vi "SetupDefault.vi"(8 "error in (no error)":errorcluster, 10 "Alias":string, 11 "SpecA_ESA in":refnum<class "SpecA_ESA.lvclass">) -> (0 "error out":errorcluster, 3 "SpecA_ESA out":refnum<class "SpecA_ESA.lvclass">)   [LabVIEW 2014, in "SpecA_ESA.lvclass"]
uses:
  SpecA_ESA.lvclass
  SpecA_ESA.lvclass/SpecA_ESA.ctl
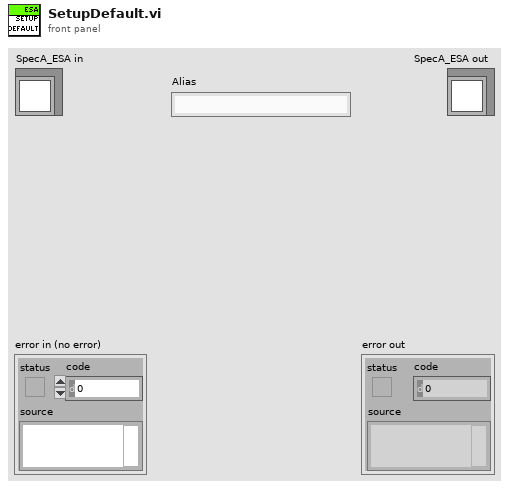
[diagram p1: front panel]
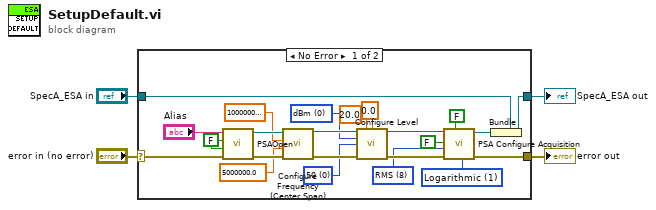
[diagram p0: block diagram]
diagram:
  n1 = case shown="No Error" "error in (no error)" {
    selector: "error in (no error)" -> [w20 w29]
    tunnel: "SpecA_ESA in" -> [w24 w28]
    tunnel: [w23 w28] -> w2
    tunnel: [w21 w29] -> w1
    frame No Error {
      w6 = 8 items=["Average", "Peak", "Sample", "Negative peak", "Quasi Peak", "EMI Average", "EMI Peak", "MIL Peak", "RMS"] ("Manual Detector Type")
      w11 = u16 0 items=["50", "75"] ("Input Impedance")
      w12 = u16 0 items=["dBm", "dBmV", "dBmA", "dBuV", "dBuVm", "dBuA", "dBuAm", "dBpt", "dBg", "Volts", "Watts", "Amps"] ("Amplitude Units")
      w26 = 1 items=["Linear", "Logarithmic"] ("Vertical Scale (0: Linear)")
      w19 = FALSE ("Calibrate Now?")
      n2 = call "PSAOpen.vi"("error in (no error)"=w20, "External CLK Ref? (True)"=w19, "Calibrate Now? (True)"=w19, "PSA In"="Alias") -> ("error out"=w18:errorcluster, "PSA Out"=w17:refnum<visa-resource-name>)  [unwired: 6 in]
      n3 = call "Configure Frequency (Center Span).vi"("error in (no error)"=w18, "Span (2 GHz)"=5000000.0 ("Center Frequency (2 GHz)"), "Center Frequency (2 GHz)"=1000000000.0, "VISA resource name"=w17) -> ("error out"=w16:errorcluster, "VISA resource name out"=w15:refnum<visa-resource-name>)  [unwired: 6 in]
      n4 = call "Configure Level.vi"("VISA resource name"=w15, "Reference Level (dBm)"=20.0, "Reference Level Offset (dB)"=0.0, "Amplitude Units"=w12, "Input Impedance"=w11, "error in (no error)"=w16) -> ("VISA resource name out"=w14:refnum<visa-resource-name>, "error out"=w13:errorcluster)  [unwired: 8 in]
      n5 = call "PSA Configure Acquisition.vi"("Vertical Scale (0: Linear)"=w26, "Enable Continuous Sweep Mode"=FALSE ("Enable Continuous Sweep Mode (F: Disable)"), "error in (no error)"=w13, "Manual Detector Type"=w6, "Enable Auto Detector"=FALSE, "VISA Refnum in"=w14) -> ("error out"=w21:errorcluster, "VISA Refnum out"=w22:refnum<visa-resource-name>)  [unwired: 4 in]
      n6 = Bundle(cluster=w24, w22) -> (w23:refnum<class "SpecA_ESA.lvclass">)
    }
    frame Error {
    }
  }
  "error out" <- w1
  "SpecA_ESA out" <- w2
